vi "Default Settings.vi"() -> (3 "Default Settings":T1={"Signal Type"=enum."Sine Wave", "Calibration Array"=[], "Log File Base Path"=path "", "EEG Channels"={"16 EEG Channels"=[], "Gain"=24}, "Soft Trig enum"=enum."Disable Soft Trigger", "Montage selection"={"Montages Ref"=refnum, "Selected Montage Number"=0, "Montages Names"=[]}, "LSL En enum"=enum."LSL Disabled"} {"EEG Channels"."16 EEG Channels"."Channel No" step=1})   [LabVIEW 2016, in "Settings Editor.lvlib"]
doc: "_____\nBased on DQMH Project Template 6.1.0.94."
uses:
  Settings Editor.lvlib
  Settings--cluster.ctl
  Acquisition/Signal Type--enum.ctl
  Acquisition/Calibration Values--cluster.ctl
  CML Shared/EEG Channel Settings.ctl
  <vilib>/Utility/sysdir.llb/System Directory Type.ctl
  Acquisition/Acquisition.lvlib
  CML Shared/CML Shared.lvlib
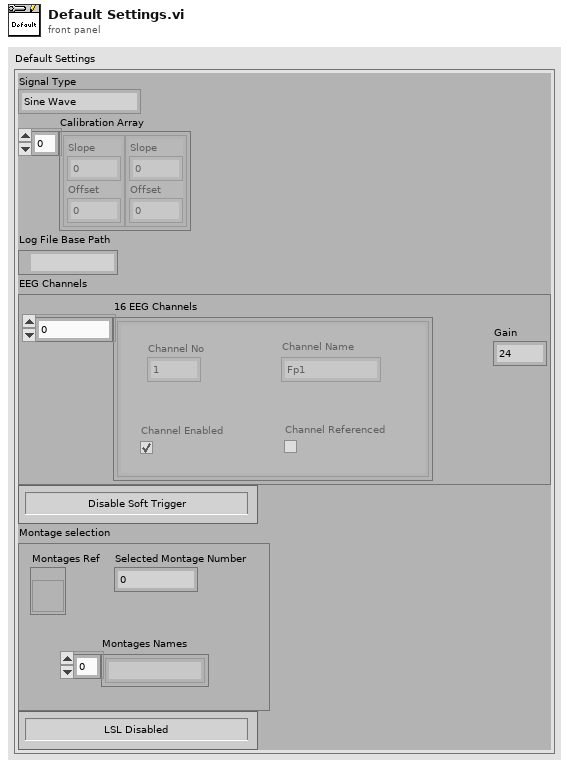
[diagram p1: front panel]
types:
  T1 = typedef "Settings Editor.lvlib/Settings--cluster.ctl" = cluster{"Signal Type":T2, "Calibration Array":T3[], "Log File Base Path":path, "EEG Channels":T4, "Soft Trig enum":enum16{"Disable Soft Trigger", "Enable Soft Trigger"}, "Montage selection":cluster{"Montages Ref":refnum<vi>, "Selected Montage Number":u8, "Montages Names":string[]}, "LSL En enum":enum16{"LSL Disabled", "LSL Enabled"}}
  T2 = typedef "Acquisition.lvlib/Signal Type--enum.ctl" = enum16{"Sine Wave", "Square with Noise"}
  T3 = typedef "Acquisition.lvlib/Calibration Values--cluster.ctl" = cluster{"Slope":dbl, "Offset":dbl}
  T4 = typedef "CML Shared.lvlib/EEG Channel Settings.ctl" = cluster{"16 EEG Channels":cluster{"Channel Name":string, "Channel No":u8, "Channel Enabled":bool, "Channel Referenced":bool}[], "Gain":u8}
  T5 = typedef "System Directory Type.ctl" = i32
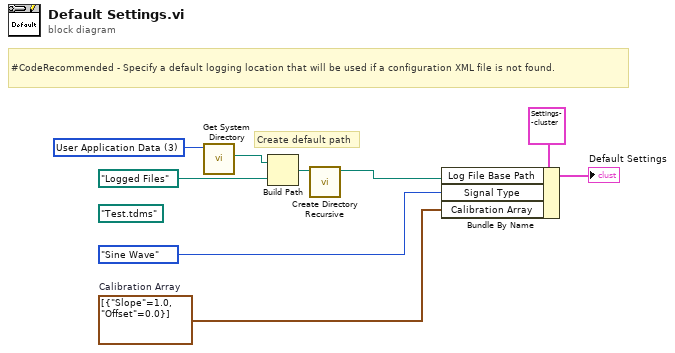
[diagram p0: block diagram]
diagram:
  (unwired) path "Test.tdms"
  w3 = T3[] [{"Slope"=1.0, "Offset"=0.0}]  # Calibration Array
  w9 = T5 3 items=["User Home"=0, "User Desktop"=1, "User Documents"=2, "User Application Data"=3, "User Preferences"=4, "User Temporary"=5, "Public Documents"=6, "Public Application Data"=7, "Public Preferences"=8, "Public Cache"=13, "System Core Libraries"=9, "System Installed Libraries"=10, "Application Files"=11, "Boot Volume Root"=12] ("system directory type")
  # "#CodeRecommended - Specify a default logging location that will be used if a configuration XML file is not found."
  # "Create default path"
  n1 = call <vilib>:"Get System Directory.vi"("system directory type"=w9) -> ("system directory"=w8:path)  [unwired: 10 in]
  n2 = Build Path(base path=w8, name or relative path=path "Logged Files") -> (appended path=w7:path)
  n3 = call <vilib>:"Create Directory Recursive.vi"("directory"=w7) -> ("directory copy"=w1:path)  [unwired: 4 in, 2 out]
  n4 = Bundle By Name(cluster=T1 {"Signal Type"=enum."Sine Wave", "Calibration Array"=[{"Slope"=1.0, "Offset"=0.0}], "Log File Base Path"=path "", "EEG Channels"={"16 EEG Channels"=[], "Gain"=24}, "Soft Trig enum"=enum."Disable Soft Trigger", "Montage selection"={"Montages Ref"=refnum, "Selected Montage Number"=0, "Montages Names"=[]}, "LSL En enum"=enum."LSL Disabled"} ("Default Settings"), "Log File Base Path"=w1, "Signal Type"=Signal_Type--enum."Sine Wave", "Calibration Array"=w3) -> (→"Default Settings":T1)
